vi "Main.vi"() -> ()   [LabVIEW 2016, in "LVJSON Tests.lvlib"]
uses:
  LVJSON Tests.lvlib
  Source/JSON Data Classes/JSON Helper/Parsing/Parse Value.vi
  Source/JSON Data Classes/JSON Datatype/JSON Null.lvclass
  Source/JSON Data Classes/JSON Helper/JSON Helper.lvclass
panel:
  out "Array":T1(array[cluster])
  # "y_structure_whitespace_array.json"
  # "Empty keys"
  # "escape characters"
  # "y_string_unicode.json"
  # "unicode"
  # "y_string_uescaped_newline.json"
  # "UTF-8"
  # "y_string_unicode_U+2064_invisible_plus.json"
  # "y_string_unicode_U+200B_ZERO_WIDTH_SPACE.json"
  # "y_string_accepted_surrogate_pair"
  # "y_string_unicode_U+1FFFE_nonchar.json"
  # "y_string_uEscape.json"
  # "y_string_unicode_escaped_double_quote.json"
  # "y_string_accepted_surrogate_pairs"
  # "y_string_backslash_and_u_escaped_zero.json"
  # "y_string_simple_ascii.json"
  # "y_string_escaped_control_character.json"
  # "y_string_surrogates_U+1D11E_MUSICAL_SYMBOL_G_CLEF.json"
  # "[\"new\\u00A0line\"]"
  # "y_string_three-byte-utf-8.json"
  # "y_string_null_escape.json"
  # "y_string_one-byte-utf-8.json"
  # "y_string_two-byte-utf-8.json"
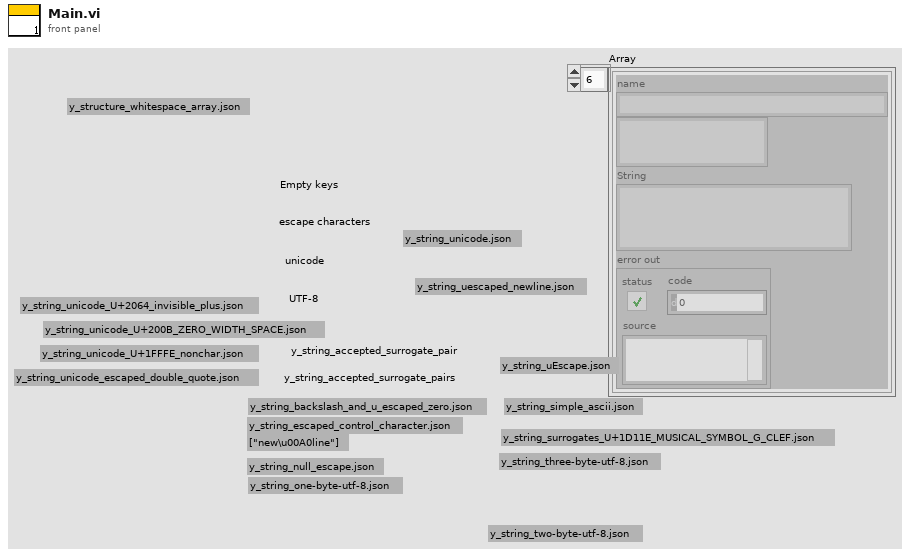
[diagram p1: front panel]
types:
  T1 = cluster{"name":string, string, "String":string, "error out":errorcluster}[]
  T2 = cluster{"name":string, string, "String":string, "error out":errorcluster}
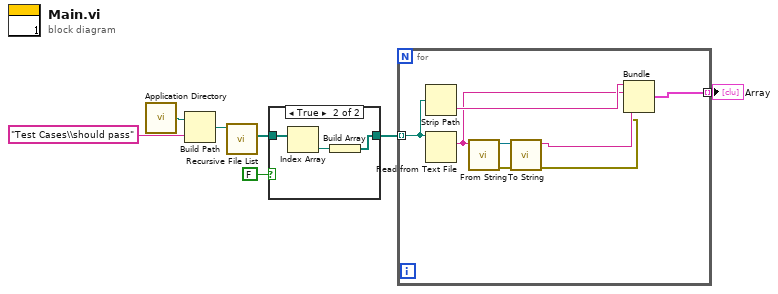
[diagram p0: block diagram]
diagram:
  n1 = call <vilib>:"Application Directory.vi"() -> ("Application Directory"=w7:path)
  n2 = Build Path(base path=w7, name or relative path="Test Cases\\should pass") -> (appended path=w5:path)
  n3 = call <vilib>:"Recursive File List.vi"("Folder Path"=w5) -> ("All Files in Dir"=w4:path[])  [unwired: 6 in, 4 out]
  n4 = case shown="True" FALSE {
    tunnel: w4 -> [w8 w11]
    tunnel: [w8 w9] -> w3
    frame False {
    }
    frame True {
      n5 = Index Array(array=w11) -> (element=w10:path)  [unwired: 1 in]
      n6 = Build Array(w10) -> (w9:path[])
    }
  }
  n7 = for {
    tunnel: w3 -> [w19] mode=indexing
    tunnel: [w15] -> w1 mode=indexing
    n8 = Strip Path(path=w19) -> (name=w17:string)  [unwired: 1 out]
    n9 = Read from Text File(file (use dialog)=w19) -> (text=w12:string)  [unwired: 3 in, 3 out]
    n10 = call "From String.vi"("JSON String"=w12) -> ("error out"=w14:errorcluster, "JSON out"=w18:refnum<class "JSON Null.lvclass">)  [unwired: 9 in]
    n11 = call-dynamic "To String.vi"("error in (no error)"=w14, "JSON Datatype in"=w18) -> ("error out"=w13:errorcluster, "String"=w16:string)  [unwired: 8 in]
    n12 = Bundle("name"=w17, w12, "String"=w16, "error out"=w13) -> (w15:T2)  [unwired: 1 in]
  }
  "Array" <- w1
